vi "Assignment 1.vi"() -> ()   [LabVIEW 2018]
panel:
  out "?":string
  in  "OK Button":bool
  out "Output":dbl
  in  "Input 2":dbl
  in  "Input 1":dbl
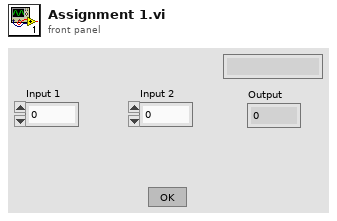
[diagram p1: front panel]
types:
  T1 = enum16{"", "None", "Add", "Sub", "Mul", "Div", "Square", "Square root", "Average", "Maximum", "Minimum"}
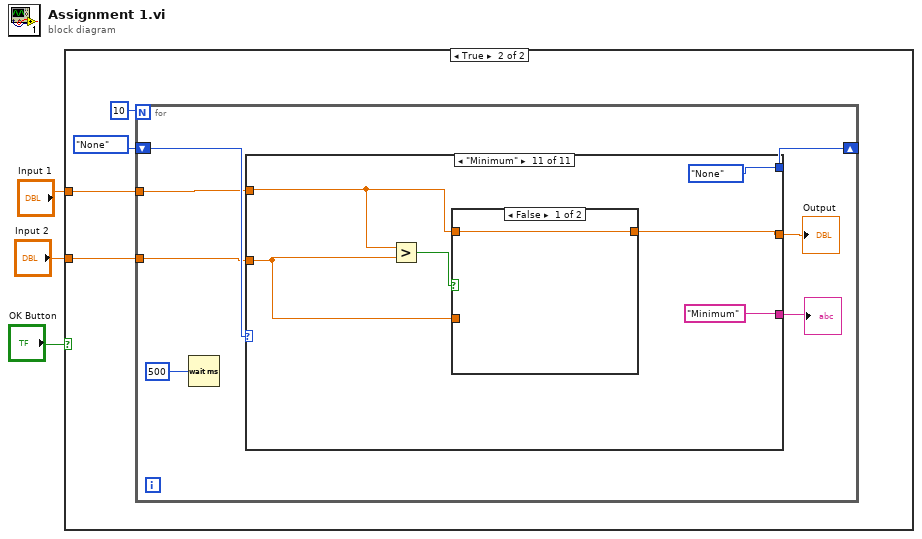
[diagram p0: block diagram]
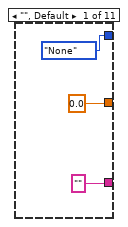
[diagram p3: hidden frame]
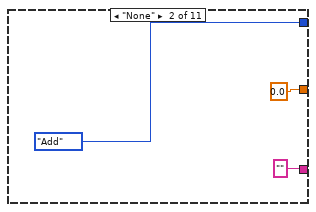
[diagram p4: hidden frame]
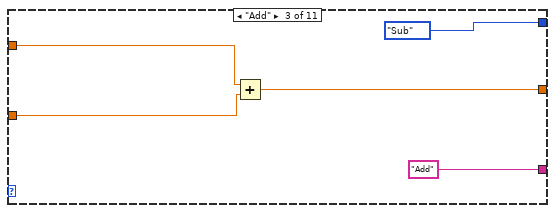
[diagram p5: hidden frame]
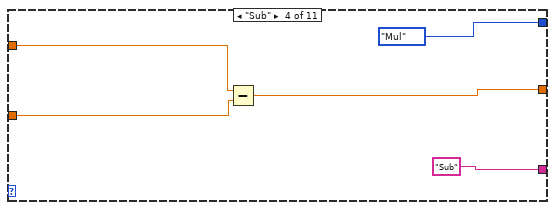
[diagram p6: hidden frame]
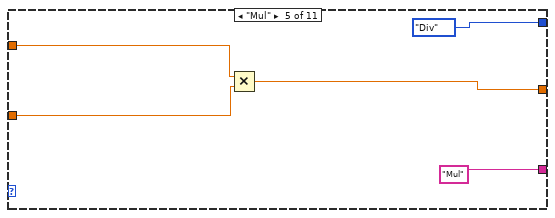
[diagram p7: hidden frame]
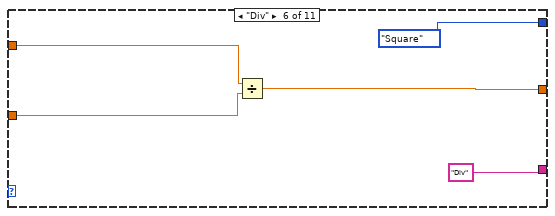
[diagram p8: hidden frame]
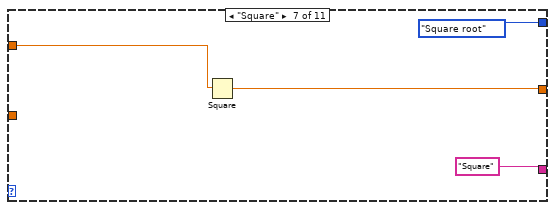
[diagram p9: hidden frame]
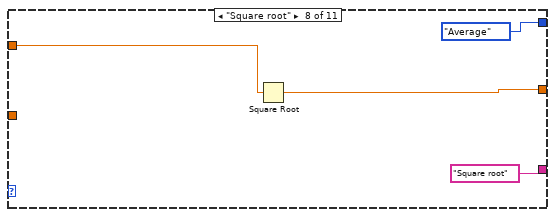
[diagram p10: hidden frame]
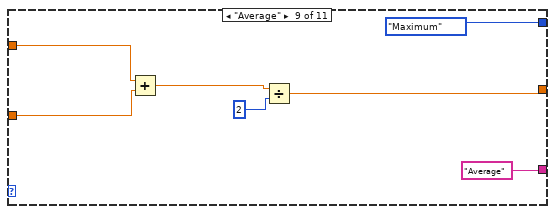
[diagram p11: hidden frame]
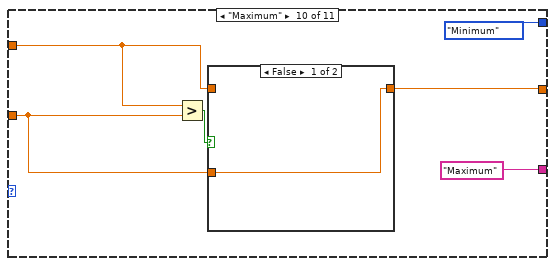
[diagram p12: hidden frame]
diagram:
  n1 = case shown="True" "OK Button" {
    tunnel: "Input 1" -> [_ w6]
    tunnel: "Input 2" -> [_ w5]
    frame False {
    }
    frame True {
      n2 = for {
        N: 10 -> [_]
        shift-right: [w13] -> _
        shift-left: T1."None" -> [w14]
        tunnel: w6 -> [w12]
        tunnel: w5 -> [w11]
        n3 = Wait (ms)(milliseconds to wait=500) -> ()  [unwired: 1 out]
        n4 = case shown="\"Minimum\"" w14 {
          tunnel: [T1."None" T1."Add" T1."Sub" T1."Mul" T1."Div" T1."Square" T1."Square root" T1."Average" T1."Maximum" T1."Minimum" T1."None"] -> w13
          tunnel: w12 -> [_ _ w24 w29 w35 w40 w44 w48 w55 w60 w68]
          tunnel: w11 -> [_ _ w23 w28 w34 w39 _ _ w54 w59 w67]
          tunnel: ["" "" "Add" "Sub" "Mul" "Div" "Square" "Square root" "Average" "Maximum" "Minimum"] -> w8
          tunnel: [0.0 0.0 w22 w27 w33 w38 w43 w47 w51 w58 w66] -> w9
          frame "", Default {
          }
          frame "None" {
          }
          frame "Add" {
            n5 = Add(x=w24, y=w23) -> (x+y=w22:dbl)
          }
          frame "Sub" {
            n6 = Subtract(x=w29, y=w28) -> (x-y=w27:dbl)
          }
          frame "Mul" {
            n7 = Multiply(x=w35, y=w34) -> (x*y=w33:dbl)
          }
          frame "Div" {
            n8 = Divide(x=w40, y=w39) -> (x/y=w38:dbl)
          }
          frame "Square" {
            n9 = Square(x=w44) -> (x^2=w43:dbl)
          }
          frame "Square root" {
            n10 = Square Root(x=w48) -> (sqrt(x)=w47:dbl)
          }
          frame "Average" {
            n11 = Add(x=w55, y=w54) -> (x+y=w53:dbl)
            n12 = Divide(x=w53, y=2) -> (x/y=w51:dbl)
          }
          frame "Maximum" {
            n13 = Greater?(x=w60, y=w59) -> (0:w61:bool)
            n14 = case shown="False" w61 {
              tunnel: w60 -> [_ w63]
              tunnel: w59 -> [w62 _]
              tunnel: [w62 w63] -> w58
              frame False {
              }
              frame True {
              }
            }
          }
          frame "Minimum" {
            n15 = Greater?(x=w68, y=w67) -> (0:w69:bool)
            n16 = case shown="False" w69 {
              tunnel: w68 -> [w70 _]
              tunnel: w67 -> [_ w71]
              tunnel: [w70 w71] -> w66
              frame False {
              }
              frame True {
              }
            }
          }
        }
        "Output" <- w9
        "?" <- w8
      }
    }
  }
